vi "Recursive File List.vi"(4 "Folders to Exclude":refnum<class "UTF-8 String.lvclass">[](array[class]), 6 "pattern":string, 8 "error in (no error)":errorcluster, 9 "Continue Recursing on Error? (F)":bool, 10 "Treat LLBs as Folders?":bool, 11 "Folder Path":refnum<class "UTF-8 Path.lvclass">) -> (0 "error out":errorcluster, 1 "Number of Files":i32, 2 "All Files in Dir":refnum<class "UTF-8 Path.lvclass">[](array[class]), 3 "dup Folder Path":refnum<class "UTF-8 Path.lvclass">, 5 "All Folders":refnum<class "UTF-8 Path.lvclass">[](array[class]))   [LabVIEW 2020, in "G-Unicode.lvlib"]
doc: "Lists the contents of a folder or LLB."
uses:
  G-Unicode.lvlib
  Types/UTF-8 Path/UTF-8 Path.lvclass
  Types/UTF-8 String/UTF-8 String.lvclass
  Types/UTF-8 String/UTF-8 String.lvclass/UTF-8 String.ctl
  Types/UTF-8 Path/UTF-8 Path.lvclass/UTF-8 Path.ctl
  d8f6ae1f-7202-4db9-b87a-1f416505b7ed.vi
  e59fd3ad-a218-449e-bbf4-8568d0899d6e.vi
  6e4bb66e-265d-408c-9dfe-e7c3a7878e52.vi
  1a260ccf-0fcf-4512-9955-37eb4df972bd.vi
  834b37ec-ea56-4ab6-91df-72f1b46fdc84.vi
  6fa5a26c-1560-4505-aaec-6e2724b388c6.vi
  de5ffccb-91e6-4fa2-acea-7dcb8ac76bcd.vi
  3afc9dd8-07d7-4035-8615-071e8f5e5c27.vi
  6eb3c72c-ccaf-45c3-aa0c-9c92d51b379f.vi
  Private/Library/gu_to_lower_case.vi
  Private/Conversion/String as Encoded String.vi
  Private/Conversion/Polymorphic VIs/String as Encoded String (UTF-8 String).vi
  Types/UTF-8 String/Write Encoded UTF-8 String.vi
  Types/UTF-8 Path/Write Encoded UTF-8 Path.vi
  Private/Conversion/Path as Encoded Path.vi
  Private/Conversion/Polymorphic VIs/Path as Encoded Path (UTF-8 Path).vi
  Path to Short Name.vi/f844562b-b612-4fa1-b092-3cf87b2107aa.vi
  Types/UTF-8 String/Read Encoded UTF-8 String.vi
  1a260ccf-0fcf-4512-9955-37eb4df972bd.vi/d1f4a45d-6f02-44dd-a40b-2b28d80e6519.vi
  1a260ccf-0fcf-4512-9955-37eb4df972bd.vi/83bb9e08-facb-42b9-b1eb-65898ec7dabd.vi
  834b37ec-ea56-4ab6-91df-72f1b46fdc84.vi/d1f4a45d-6f02-44dd-a40b-2b28d80e6519.vi
  834b37ec-ea56-4ab6-91df-72f1b46fdc84.vi/83bb9e08-facb-42b9-b1eb-65898ec7dabd.vi
  6fa5a26c-1560-4505-aaec-6e2724b388c6.vi/4d3f9d4a-5006-44fd-9ac3-fe6a2ce0b86b.vi
  6fa5a26c-1560-4505-aaec-6e2724b388c6.vi/29e5914f-c0b0-4539-b998-9919647c2bfd.vi
  de5ffccb-91e6-4fa2-acea-7dcb8ac76bcd.vi/4d3f9d4a-5006-44fd-9ac3-fe6a2ce0b86b.vi
  de5ffccb-91e6-4fa2-acea-7dcb8ac76bcd.vi/29e5914f-c0b0-4539-b998-9919647c2bfd.vi
  Private/Conversion/Text as Encoded Path.vi
  Private/Conversion/Polymorphic VIs/Text as Encoded Path (UTF-8 String).vi
  Types/UTF-8 Path/Read Encoded UTF-8 Path.vi
  Private/Conversion/Text as Encoded String.vi
  Private/Conversion/Polymorphic VIs/Text as Encoded String (UTF-8 Path).vi
  Private/Conversion/Polymorphic VIs/Text as Encoded String (UTF-8 String).vi
  Private/Conversion/Polymorphic VIs/Text as Encoded String (LabVIEW String).vi
  Unicode/Encoded UTF-8 String to Encoded UTF-16LE String.vi
  Unicode/Encoded UTF-16LE String to Encoded UTF-8 String.vi
  Private/Memory/Copy String Array.vi
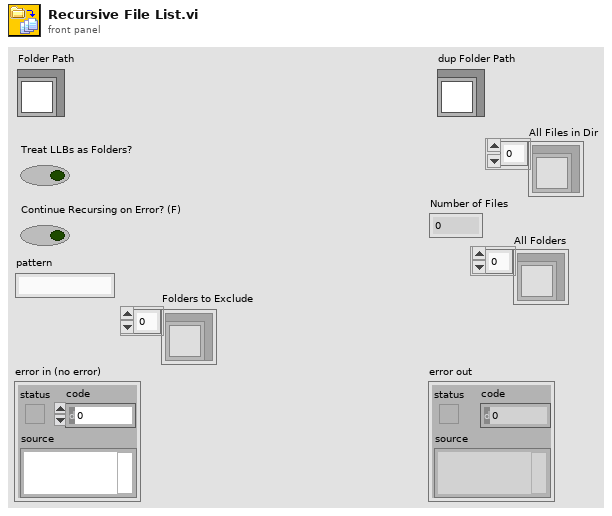
[diagram p1: front panel]
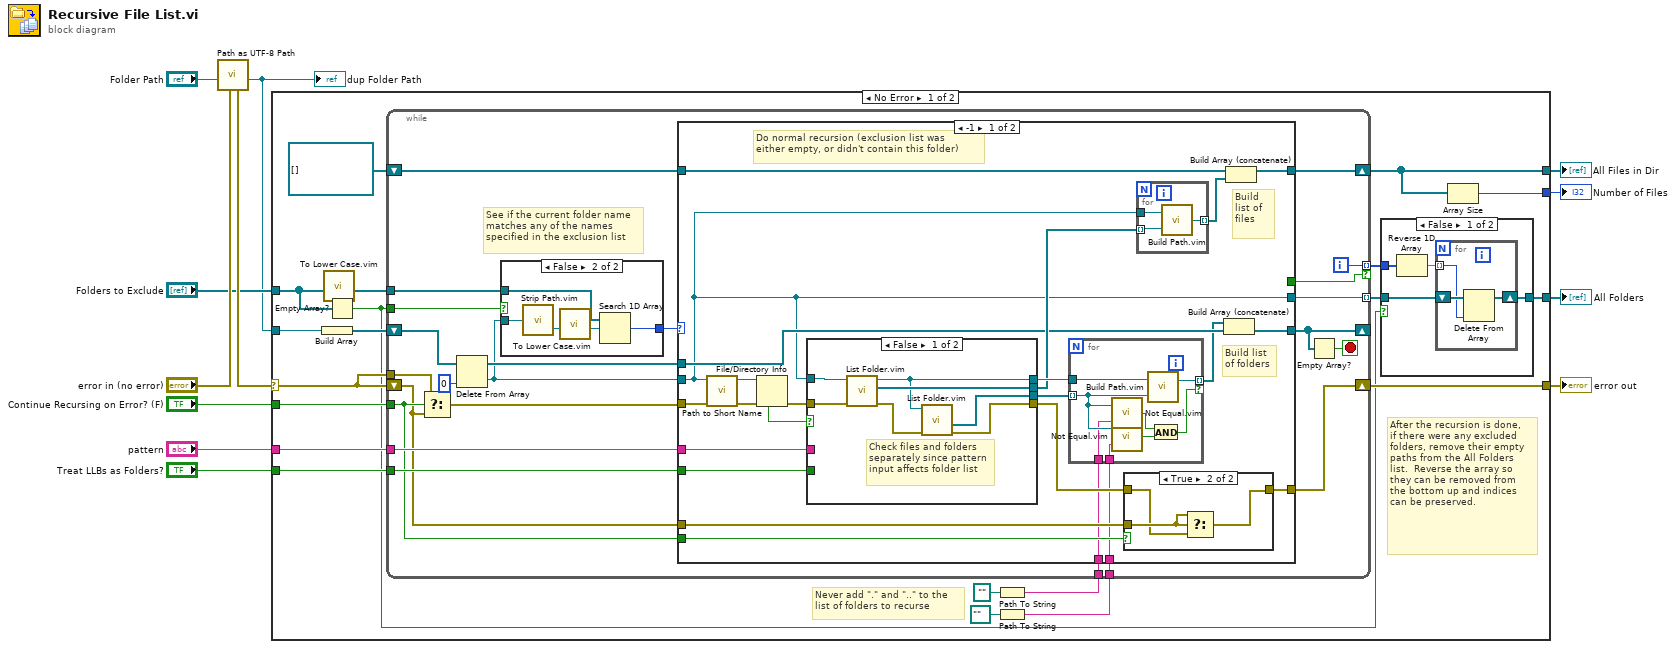
[diagram p0: block diagram]
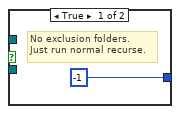
[diagram p2: hidden frame]
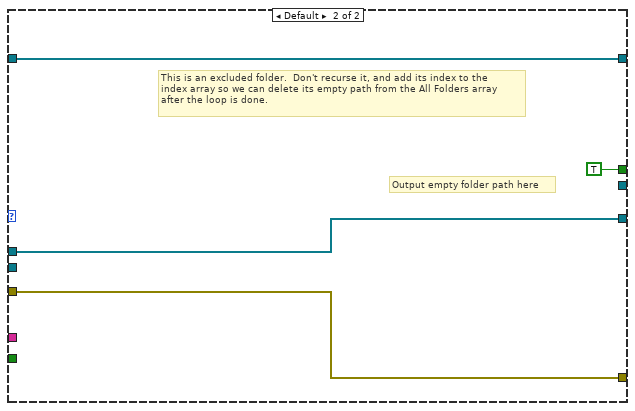
[diagram p5: hidden frame]
diagram:
  n1 = call "Path as UTF-8 Path.vi"("error in"="error in (no error)", "Path"="Folder Path") -> ("UTF-8 Path"=w2:refnum<class "UTF-8 Path.lvclass">, "error out"=w11:errorcluster)  [unwired: 8 in]
  "dup Folder Path" <- w2
  n2 = case shown="No Error" w11 {
    selector: w11 -> [w23 w121]
    tunnel: w2 -> [w32 _]
    tunnel: [w26 _] -> w10
    tunnel: [w25 _] -> w9
    tunnel: [w27 w121] -> w8
    tunnel: "Treat LLBs as Folders?" -> [w29 _]
    tunnel: [w20 _] -> w6
    tunnel: "pattern" -> [w28 _]
    tunnel: "Continue Recursing on Error? (F)" -> [w24 _]
    tunnel: "Folders to Exclude" -> [w13 _]
    frame No Error {
      # "Never add \".\" and \"..\" to the list of folders to recurse"
      # "After the recursion is done,\nif there were any excluded\nfolders, remove their empty\npaths from the All Folders\nlist.  Reverse the array so\nthey can be removed from\nthe bottom up and indices\ncan be preserved."
      n3 = Build Array(w32) -> (w31:refnum<class "UTF-8 Path.lvclass">[])
      n4 = call "To Lower Case.vim"("String"=w13) -> ("All Lower Case String"=w22:refnum<class "UTF-8 String.lvclass">[])  [unwired: 9 in, 1 out]
      n5 = Empty Array?(array=w13) -> (empty?=w18:bool)
      n6 = Path To String(path=path "") -> (string=w15:string)
      n7 = Path To String(path=path "..") -> (string=w14:string)
      n8 = while {
        shift-left: refnum<class "UTF-8 Path.lvclass">[] [] ("Array Constant") -> [w53]
        shift-right: [w55] -> w26
        shift-left: w31 -> [w54]
        shift-right: [w50] -> _
        shift-right: [w44] -> w27
        shift-left: w23 -> [w43]
        tunnel: w29 -> [w52]
        tunnel: [w41] -> w21 mode=indexing
        tunnel: w28 -> [w51]
        tunnel: w24 -> [w45]
        tunnel: w23 -> [w46]
        tunnel: w22 -> [w39]
        tunnel: w18 -> [w40]
        tunnel: [w36] -> w19 mode=indexing if=w35
        tunnel: w15 -> [w34]
        tunnel: w14 -> [w33]
        i -> [w36]
        stop <- w49 stop-if-true
        # "See if the current folder name\nmatches any of the names\nspecified in the exclusion list"
        n9 = Select(t=w46, s=w45, f=w43) -> (s? t:f=w47:errorcluster)
        n10 = Delete From Array(array=w54, index=0) -> (deleted portion=w38:refnum<class "UTF-8 Path.lvclass">, array with subset deleted=w42:refnum<class "UTF-8 Path.lvclass">[])  [unwired: 1 in]
        n11 = case shown="False" w40 {
          tunnel: w39 -> [_ w59]
          tunnel: w38 -> [_ w61]
          tunnel: [-1 ("index of element") w58] -> w37
          frame True {
            # "No exclusion folders.\nJust run normal recurse."
          }
          frame False {
            n12 = call "Strip Path.vim"("Path"=w61) -> ("Name"=w57:refnum<class "UTF-8 String.lvclass">)  [unwired: 1 out]
            n13 = call "To Lower Case.vim"("String"=w57) -> ("All Lower Case String"=w60:refnum<class "UTF-8 String.lvclass">)  [unwired: 9 in, 1 out]
            n14 = Search 1D Array(1D array=w59, element=w60) -> (index of element=w58:i32)  [unwired: 1 out]
          }
        }
        n15 = case shown="-1" w37 {
          tunnel: [w84 w112] -> w55
          tunnel: w53 -> [w83 w112]
          tunnel: w52 -> [w81 _]
          tunnel: w51 -> [w80 _]
          tunnel: [w78 w111] -> w50
          tunnel: w38 -> [w62 _]
          tunnel: w47 -> [w64 w110]
          tunnel: w45 -> [w74 _]
          tunnel: [w73 w110] -> w44
          tunnel: w43 -> [w72 _]
          tunnel: w42 -> [w70 w111]
          tunnel: [w62 _] -> w41
          tunnel: [_ TRUE] -> w35
          tunnel: w34 -> [w67 _]
          tunnel: w33 -> [w66 _]
          frame -1 {
            # "Build list of files"
            # "Build list\nof folders"
            # "Do normal recursion (exclusion list was\neither empty, or didn't contain this folder)"
            n16 = call "Path to Short Name.vi"("error in"=w64, "Path"=w62) -> ("error out"=w63:errorcluster, "LabVIEW Path"=w65:path)  [unwired: 8 in]
            n17 = File/Directory Info(path=w65, error in=w63) -> (error out=w77:errorcluster, shortcut=w76:bool)  [unwired: 5 out]
            n18 = case shown="False" w76 {
              tunnel: [w99 _] -> w71
              tunnel: [w98 w101] -> w82
              tunnel: [w97 w100] -> w75
              tunnel: w81 -> [_ _]
              tunnel: w80 -> [_ _]
              tunnel: [w96 _] -> w79
              tunnel: w77 -> [w95 w100]
              tunnel: w62 -> [w94 w101]
              frame False {
                # "Check files and folders\nseparately since pattern\ninput affects folder list"
                n19 = call "List Folder.vim"("error in"=w95, "Path"=w94) -> ("error out"=w93:errorcluster, "Filenames"=w99:refnum<class "UTF-8 String.lvclass">[], "Path Out"=w98:refnum<class "UTF-8 Path.lvclass">)  [unwired: 6 in, 1 out]
                n20 = call "List Folder.vim"("error in"=w93, "Path"=w98) -> ("error out"=w97:errorcluster, "Folder Names"=w96:refnum<class "UTF-8 String.lvclass">[])  [unwired: 6 in, 2 out]
              }
              frame True {
                # "Do not attempt to recurse the contents of folder shortcuts"
              }
            }
            n21 = for {
              tunnel: w82 -> [w92]
              tunnel: [w91] -> w69 mode=indexing if=w90
              tunnel: w79 -> [w89] mode=indexing
              tunnel: w67 -> [w88]
              tunnel: w66 -> [w87]
              n22 = call "Not Equal.vim"("y"=w88, "x"=w89) -> ("Not Equal?"=w85:bool)
              n23 = call "Not Equal.vim"("y"=w87, "x"=w89) -> ("Not Equal?"=w86:bool)
              n24 = call "Build Path.vim"("Name or Relative Path"=w89, "Base Path"=w92) -> ("Appended Path"=w91:refnum<class "UTF-8 Path.lvclass">)
              n25 = And(x=w85, y=w86) -> (x .and. y?=w90:bool)
            }
            n26 = case shown="True" w74 {
              tunnel: w75 -> [w105 w107]
              tunnel: [w105 w106] -> w73
              tunnel: w72 -> [_ w108]
              frame False {
              }
              frame True {
                n27 = Select(t=w108, s=w108, f=w107) -> (s? t:f=w106:errorcluster)
              }
            }
            n28 = for {
              tunnel: w71 -> [w103] mode=indexing
              tunnel: w62 -> [w104]
              tunnel: [w102] -> w68 mode=indexing
              n29 = call "Build Path.vim"("Name or Relative Path"=w103, "Base Path"=w104) -> ("Appended Path"=w102:refnum<class "UTF-8 Path.lvclass">)
            }
            n30 = Build Array (concatenate)(w69, w70) -> (w78:refnum<class "UTF-8 Path.lvclass">[])
            n31 = Build Array (concatenate)(w83, w68) -> (w84:refnum<class "UTF-8 Path.lvclass">[])
          }
          frame Default {
            # "Output empty folder path here"
            # "This is an excluded folder.  Don't recurse it, and add its index to the\nindex array so we can delete its empty path from the All Folders array\nafter the loop is done."
          }
        }
        n32 = Empty Array?(array=w50) -> (empty?=w49:bool)
      }
      n33 = case shown="False" w18 {
        tunnel: w21 -> [w115 w120]
        tunnel: [w114 w120] -> w20
        tunnel: w19 -> [w116 _]
        frame False {
          n34 = Reverse 1D Array(array=w116) -> (reversed array=w113:i32[])
          n35 = for {
            shift-right: [w118] -> w114
            shift-left: w115 -> [w119]
            tunnel: w113 -> [w117] mode=indexing
            n36 = Delete From Array(array=w119, index=w117) -> (array with subset deleted=w118:refnum<class "UTF-8 Path.lvclass">[])  [unwired: 1 in, 1 out]
          }
        }
        frame True {
          # "No excluded folders.\nDon't run the code that\ndeletes excluded folder\nindices."
        }
      }
      n37 = Array Size(array=w26) -> (size(s)=w25:i32)
    }
    frame Error {
    }
  }
  "All Files in Dir" <- w10
  "Number of Files" <- w9
  "error out" <- w8
  "All Folders" <- w6
